vi "Read (Single Response).vi"(8 "error in (no error)":errorcluster, 11 "VISA resource name":refnum<visa-resource-name>) -> (0 "error out":errorcluster, 1 "Response Bundle":T1, 2 "Response":string, 3 "VISA resource name out":refnum<visa-resource-name>)   [LabVIEW 2020, in "Zaber A Series.lvlib"]
doc: "Reads a single response from the Serial buffer. The complete string is returned on the Response output, and the details of the format of the response are described here: http://www.zaber.com/wiki/Manuals/ASCII_Protocol_Manual#Replies. This VI also parses the string, bundles the components, and returns the bundle on the Response Bundle pin. \n\nThe Response Bundle is designed to extract data from Replies only. Info and Alert type responses will not make sense in the Bundle and should be read with just the Response output. By default the only Info or Alert type responses you can expect directly follow 'help' commands. \n\nThis VI requires that the Initialize VI has been called with the same serial port. \n\nThe Data string of the response is checked for rejection responses and if any are detected will send a warning on the error out. The possible warnings are:\n\n1073481729 - BADCHECKSUM - The checksum provided in the command message was incorrect.\n1073481730 - BADCOMMAND - The command or setting is incorrect or invalid.\n1073481731 - BADDATA - The data provided in the command is incorrect or out of range.\n1073481732 - STATUSBUSY - The device cannot be parked, nor can certain settings be changed, because it is currently busy.\n1073481733 - DEVICEONLY - An axis number was specified when trying to execute a device only command.\n1073481734 - PARKED - The device cannot move because it is currently parked.\n1073481735 - AGAIN - The stream queue is full. The command should be resent until AGAIN is not received. \n1073481736 - BADMESSAGEID - A message ID was provided, but was not either -- or a number from 0 to 99.\n1073481737 - BADAXIS - The command was sent with an axis number greater than the number of axes available.\n1073481738 - LOCKSTEP - An axis cannot be moved using normal motion commands because it is part of a lockstep group. You must use lockstep commands for motion or disable the lockstep group first.\n1073481739 - FULL - The device has run out of permanent storage and cannot accept the command. Occurs when storing to a stream buffer or when saving commands to joystick keys.\n1073481740 - NOACCESS - The command or setting is not available at the current access level.\n\nNote: This VI is set to read 100 bytes, but will terminate when it sees the new line character in order to return only one response. It's assumed that responses will be shorter than 100 characters. If your responses exceed this for any reason, adjust the constant to a higher number."
uses:
  Zaber A Series.lvlib
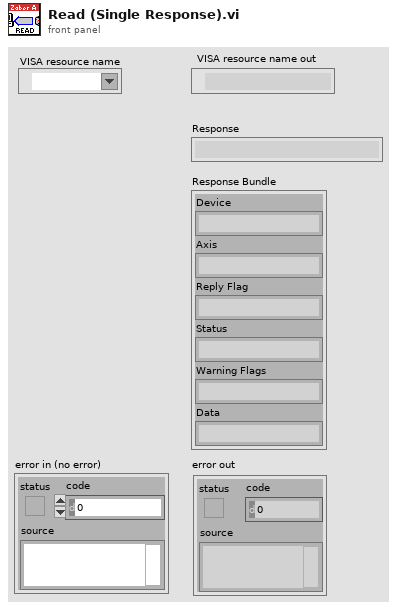
[diagram p1: front panel]
types:
  T1 = cluster{"Device":string, "Axis":string, "Reply Flag":string, "Status":string, "Warning Flags":string, "Data":string}
  T2 = cluster{string, string, string, string, string, "spreadsheet string":string}
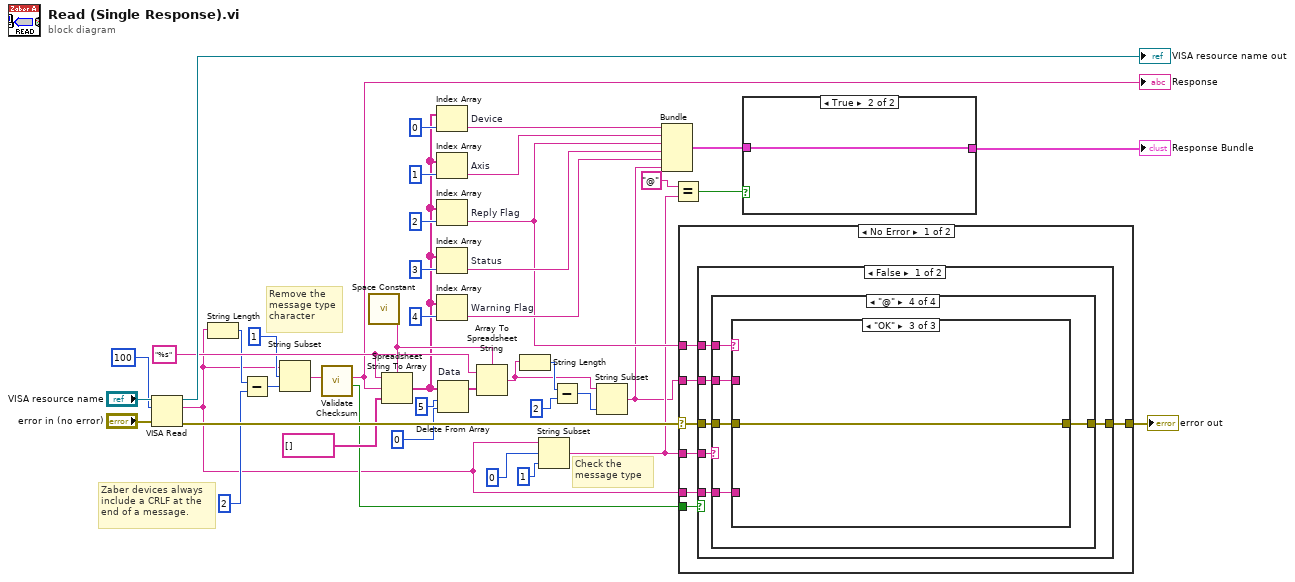
[diagram p0: block diagram]
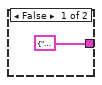
[diagram p2: hidden frame]
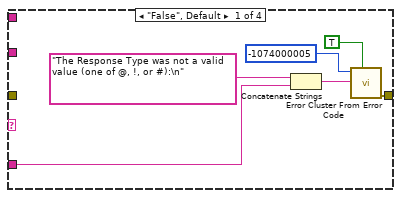
[diagram p3: hidden frame]
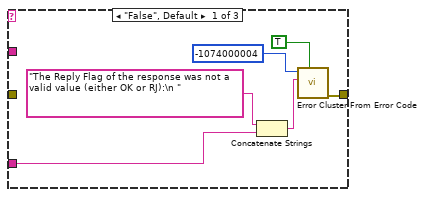
[diagram p6: hidden frame]
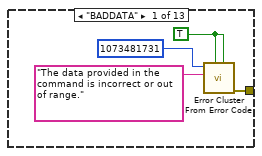
[diagram p8: hidden frame]
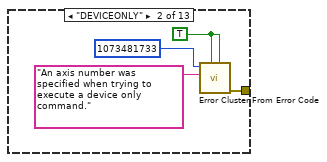
[diagram p9: hidden frame]
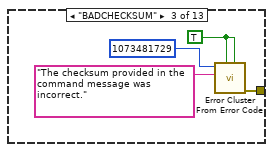
[diagram p10: hidden frame]
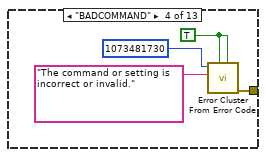
[diagram p11: hidden frame]
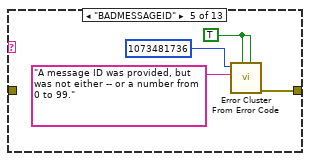
[diagram p12: hidden frame]
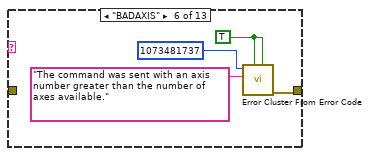
[diagram p13: hidden frame]
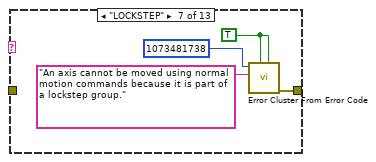
[diagram p14: hidden frame]
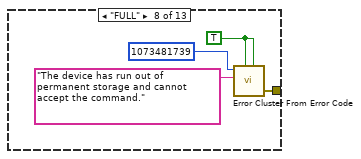
[diagram p15: hidden frame]
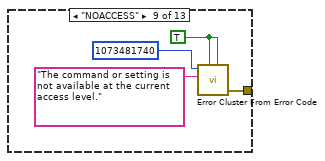
[diagram p16: hidden frame]
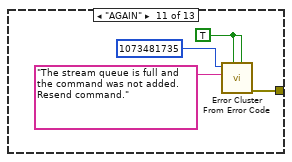
[diagram p17: hidden frame]
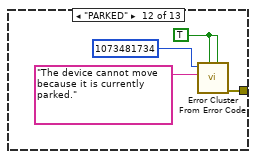
[diagram p18: hidden frame]
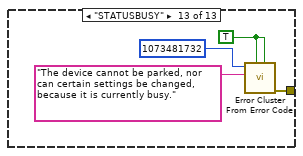
[diagram p19: hidden frame]
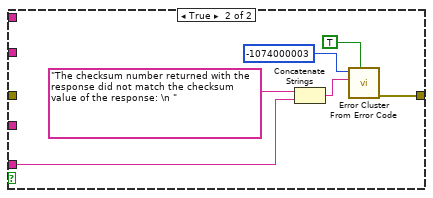
[diagram p20: hidden frame]
diagram:
  w23 = "%s" ("format string")
  # "Check the\nmessage type"
  # "Remove the \nmessage type\ncharacter"
  # "Zaber devices always \ninclude a CRLF at the\nend of a message."
  n1 = VISA Read(VISA resource name="VISA resource name", byte count=u32 100, error in (no error)="error in (no error)") -> (VISA resource name out=→"VISA resource name out":refnum<visa-resource-name>, read buffer=w11:string, error out=w39:errorcluster)  [unwired: 1 out]
  n2 = String Length(string=w11) -> (length=w17:i32)
  n3 = Subtract(x=w17, y=2) -> (x-y=w16:i32)
  n4 = String Subset(string=w11, offset (0)=1, length (rest)=w16) -> (substring=w14:string)
  n5 = call "Validate Checksum.vi"("Response"=w14) -> ("Invalid Checksum?"=w12:bool, "Remaining Response"=w13:string)  [unwired: 9 in]
  "Response" <- w13
  n6 = call <vilib>:"Space Constant.vi"() -> ("String"=w31:string)
  n7 = Spreadsheet String To Array(delimiter (Tab)=w31, format string=w23, spreadsheet string=w13, array type (2D Dbl)=string[] []) -> (array=w22:string[])
  n8 = Index Array "Device"(array=w22, index=0) -> (element=w36:string)
  n9 = Index Array "Axis"(array=w22, index=1) -> (element=w35:string)
  n10 = Index Array "Reply Flag"(array=w22, index=2) -> (element=w18:string)
  n11 = Index Array "Status"(array=w22, index=3) -> (element=w34:string)
  n12 = Index Array "Warning Flag"(array=w22, index=4) -> (element=w33:string)
  n13 = Delete From Array "Data"(array=w22, length=5, index=0) -> (array with subset deleted=w32:string[])  [unwired: 1 out]
  n14 = Array To Spreadsheet String(delimiter (Tab)=w31, array=w32, 3:w23) -> (spreadsheet string=w2:string)
  n15 = String Length(string=w2) -> (length=w4:i32)
  n16 = String Subset(string=w11, offset (0)=0, length (rest)=1 ("length (rest)")) -> (substring=w8:string)
  n17 = Subtract(x=w4, y=2) -> (x-y=w3:i32)
  n18 = String Subset(string=w2, length (rest)=w3) -> (substring=w1:string)  [unwired: 1 in]
  n19 = Bundle(w36, w35, w18, w34, w33, "spreadsheet string"=w1) -> (w10:T2)  [unwired: 1 in]
  n20 = Equal?(x="@", y=w8) -> (x = y?=w6:bool)
  n21 = case shown="No Error" w39 {
    selector: w39 -> [w48 w135]
    tunnel: [w50 w135] -> w38
    tunnel: w1 -> [w49 _]
    tunnel: w8 -> [w47 _]
    tunnel: w18 -> [w46 _]
    tunnel: w12 -> [w45 _]
    tunnel: w11 -> [w44 _]
    frame No Error {
      n22 = case shown="False" w45 {
        tunnel: [w56 w132] -> w50
        tunnel: w49 -> [w55 _]
        tunnel: w48 -> [w54 _]
        tunnel: w47 -> [w53 _]
        tunnel: w46 -> [w52 _]
        tunnel: w44 -> [w51 w130]
        frame False {
          n23 = case shown="\"@\"" w53 {
            tunnel: [w60 w63 w64 w69] -> w56
            tunnel: w55 -> [_ _ _ w68]
            tunnel: w54 -> [_ w63 w64 w67]
            tunnel: w52 -> [_ _ _ w66]
            tunnel: w51 -> [w57 _ _ w65]
            frame "False", Default {
              n24 = Concatenate Strings("The Response Type was not a valid value (one of @, !, or #):\n" ("error message (\"\")"), w57) -> (w59:string)
              n25 = call <vilib>:"Error Cluster From Error Code.vi"("show call chain? (False)"=TRUE, "error message (\"\")"=w59, "error code (0)"=-1074000005) -> ("error out"=w60:errorcluster)  [unwired: 6 in]
            }
            frame "!" {
            }
            frame "#" {
            }
            frame "@" {
              n26 = case shown="\"OK\"" w66 {
                tunnel: [w73 w78 w128] -> w69
                tunnel: w68 -> [_ w77 _]
                tunnel: w67 -> [_ w76 w128]
                tunnel: w65 -> [w72 _ _]
                frame "False", Default {
                  n27 = Concatenate Strings("The Reply Flag of the response was not a valid value (either OK or RJ):\n " ("error message (\"\")"), w72) -> (w70:string)
                  n28 = call <vilib>:"Error Cluster From Error Code.vi"("show call chain? (False)"=TRUE, "error message (\"\")"=w70, "error code (0)"=-1074000004) -> ("error out"=w73:errorcluster)  [unwired: 6 in]
                }
                frame "RJ" {
                  n29 = case shown="Default" w77 {
                    tunnel: [w79 w85 w87 w91 w95 w99 w103 w107 w111 w115 w116 w121 w125] -> w78
                    tunnel: w76 -> [_ _ _ _ _ _ _ _ _ w115 _ _ _]
                    frame "BADDATA" {
                      w82 = TRUE
                      n30 = call <vilib>:"Error Cluster From Error Code.vi"("is warning? (False)"=w82, "show call chain? (False)"=w82, "error message (\"\")"="The data provided in the command is incorrect or out of range." ("error message (\"\")"), "error code (0)"=1073481731) -> ("error out"=w79:errorcluster)  [unwired: 5 in]
                    }
                    frame "DEVICEONLY" {
                      w86 = TRUE
                      n31 = call <vilib>:"Error Cluster From Error Code.vi"("is warning? (False)"=w86, "show call chain? (False)"=w86, "error message (\"\")"="An axis number was specified when trying to execute a device only command." ("error message (\"\")"), "error code (0)"=1073481733) -> ("error out"=w85:errorcluster)  [unwired: 5 in]
                    }
                    frame "BADCHECKSUM" {
                      w90 = TRUE
                      n32 = call <vilib>:"Error Cluster From Error Code.vi"("is warning? (False)"=w90, "show call chain? (False)"=w90, "error message (\"\")"="The checksum provided in the command message was incorrect." ("error message (\"\")"), "error code (0)"=1073481729) -> ("error out"=w87:errorcluster)  [unwired: 5 in]
                    }
                    frame "BADCOMMAND" {
                      w94 = TRUE
                      n33 = call <vilib>:"Error Cluster From Error Code.vi"("is warning? (False)"=w94, "show call chain? (False)"=w94, "error message (\"\")"="The command or setting is incorrect or invalid." ("error message (\"\")"), "error code (0)"=1073481730) -> ("error out"=w91:errorcluster)  [unwired: 5 in]
                    }
                    frame "BADMESSAGEID" {
                      w98 = TRUE
                      n34 = call <vilib>:"Error Cluster From Error Code.vi"("is warning? (False)"=w98, "show call chain? (False)"=w98, "error message (\"\")"="A message ID was provided, but was not either -- or a number from 0 to 99." ("error message (\"\")"), "error code (0)"=1073481736) -> ("error out"=w95:errorcluster)  [unwired: 5 in]
                    }
                    frame "BADAXIS" {
                      w100 = TRUE
                      n35 = call <vilib>:"Error Cluster From Error Code.vi"("is warning? (False)"=w100, "show call chain? (False)"=w100, "error message (\"\")"="The command was sent with an axis number greater than the number of axes available." ("error message (\"\")"), "error code (0)"=1073481737) -> ("error out"=w99:errorcluster)  [unwired: 5 in]
                    }
                    frame "LOCKSTEP" {
                      w106 = TRUE
                      n36 = call <vilib>:"Error Cluster From Error Code.vi"("is warning? (False)"=w106, "show call chain? (False)"=w106, "error message (\"\")"="An axis cannot be moved using normal motion commands because it is part of a lockstep group." ("error message (\"\")"), "error code (0)"=1073481738) -> ("error out"=w103:errorcluster)  [unwired: 5 in]
                    }
                    frame "FULL" {
                      w108 = TRUE
                      n37 = call <vilib>:"Error Cluster From Error Code.vi"("is warning? (False)"=w108, "show call chain? (False)"=w108, "error message (\"\")"="The device has run out of permanent storage and cannot accept the command." ("error message (\"\")"), "error code (0)"=1073481739) -> ("error out"=w107:errorcluster)  [unwired: 5 in]
                    }
                    frame "NOACCESS" {
                      w114 = TRUE
                      n38 = call <vilib>:"Error Cluster From Error Code.vi"("is warning? (False)"=w114, "show call chain? (False)"=w114, "error message (\"\")"="The command or setting is not available at the current access level." ("error message (\"\")"), "error code (0)"=1073481740) -> ("error out"=w111:errorcluster)  [unwired: 5 in]
                    }
                    frame Default {
                    }
                    frame "AGAIN" {
                      w119 = TRUE
                      n39 = call <vilib>:"Error Cluster From Error Code.vi"("is warning? (False)"=w119, "show call chain? (False)"=w119, "error message (\"\")"="The stream queue is full and the command was not added. Resend command." ("error message (\"\")"), "error code (0)"=1073481735) -> ("error out"=w116:errorcluster)  [unwired: 5 in]
                    }
                    frame "PARKED" {
                      w123 = TRUE
                      n40 = call <vilib>:"Error Cluster From Error Code.vi"("is warning? (False)"=w123, "show call chain? (False)"=w123, "error message (\"\")"="The device cannot move because it is currently parked." ("error message (\"\")"), "error code (0)"=1073481734) -> ("error out"=w121:errorcluster)  [unwired: 5 in]
                    }
                    frame "STATUSBUSY" {
                      w127 = TRUE
                      n41 = call <vilib>:"Error Cluster From Error Code.vi"("is warning? (False)"=w127, "show call chain? (False)"=w127, "error message (\"\")"="The device cannot be parked, nor can certain settings be changed, because it is currently busy." ("error message (\"\")"), "error code (0)"=1073481732) -> ("error out"=w125:errorcluster)  [unwired: 5 in]
                    }
                  }
                }
                frame "OK" {
                }
              }
            }
          }
        }
        frame True {
          n42 = Concatenate Strings("The checksum number returned with the response did not match the checksum value of the response: \n " ("error message (\"\")"), w130) -> (w129:string)
          n43 = call <vilib>:"Error Cluster From Error Code.vi"("show call chain? (False)"=TRUE, "error message (\"\")"=w129, "error code (0)"=-1074000003) -> ("error out"=w132:errorcluster)  [unwired: 6 in]
        }
      }
    }
    frame Error {
    }
  }
  "error out" <- w38
  n44 = case shown="True" w6 {
    tunnel: w10 -> [_ w137]
    tunnel: [T2 {"", "", "", "", "", "spreadsheet string"=""} ("output cluster") w137] -> w9
    frame False {
    }
    frame True {
    }
  }
  "Response Bundle" <- w9
